vi "get User Info List.vi"(8 "error in (no error)":errorcluster, 11 "[Data] Userinfo Binary in":refnum<class "[Data] Userinfo Binary.lvclass">) -> (0 "error out":errorcluster, 2 "user info":T1(array[cluster]), 3 "[Data] Userinfo Binary out":refnum<class "[Data] Userinfo Binary.lvclass">)   [LabVIEW 2020, in "[Data] Userinfo Binary.lvclass"]
uses:
  [Data] Userinfo Binary.lvclass
  [Data] Userinfo Binary.lvclass/[Data] Userinfo Binary.ctl
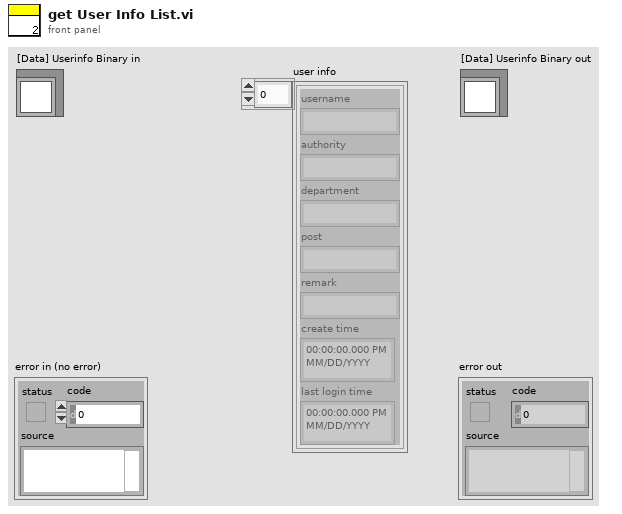
[diagram p1: front panel]
types:
  T1 = cluster{"username":string, "authority":string, "department":string, "post":string, "remark":string, "create time":timestamp, "last login time":timestamp}[]
  T2 = cluster{"username":string, "authority":string, "department":string, "post":string, "remark":string, "create time":timestamp, "last login time":timestamp}
  T3 = typedef "[Data] Userinfo Binary.lvclass/user info.ctl" = cluster{"password":string, "authority":i8, "department":string, "post":string, "remark":string, "create time":timestamp, "last login time":timestamp}
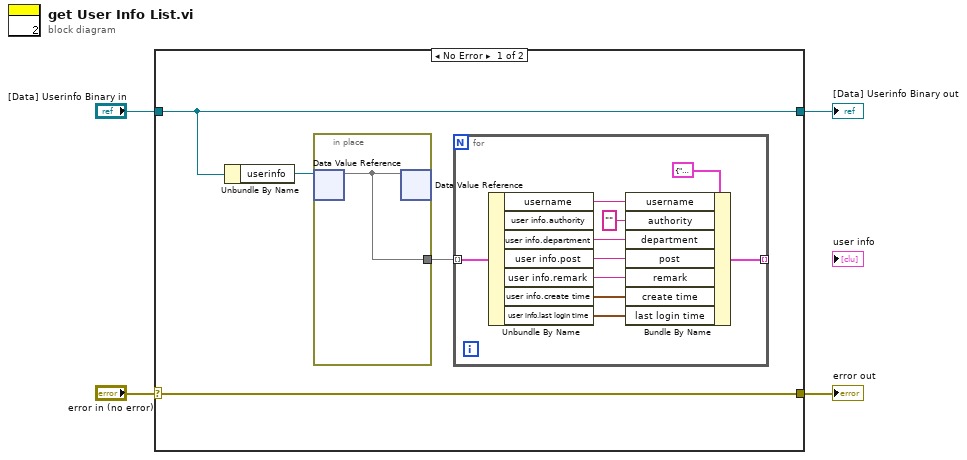
[diagram p0: block diagram]
diagram:
  n1 = case shown="No Error" "error in (no error)" {
    selector: "error in (no error)" -> [w8 w21]
    tunnel: [w8 w21] -> w1
    tunnel: "[Data] Userinfo Binary in" -> [w7 w20]
    tunnel: [w7 w20] -> w3
    frame No Error {
      n2 = Unbundle By Name(w7) -> ("userinfo"=w6:refnum<data-value>)
      n3 = in-place {
        in-place-border: [w19] -> w5
        n4 = in-place-dvr #1(w6) -> (w19:map{string, T3})  [unwired: 1 out]
        n5 = in-place-dvr #1(w19) -> ()  [unwired: 2 out]
      }
      n6 = for {
        tunnel: w5 -> [w18] mode=indexing
        tunnel: [w11] -> _ mode=indexing
        n7 = Unbundle By Name(w18) -> ("username"=w17:string, "user info.department"=w16:string, "user info.post"=w15:string, "user info.remark"=w14:string, "user info.create time"=w13:timestamp, "user info.last login time"=w12:timestamp)  [unwired: 1 out]
        n8 = Bundle By Name(cluster=T2 {"username"="admin", "authority"="", "department"="", "post"="", "remark"="", "create time"=timestamp(3808709554.2178783 s since 1904-01-01), "last login time"=timestamp(3808709806.919703 s since 1904-01-01)} ("user info"), "username"=w17, "authority"="", "department"=w16, "post"=w15, "remark"=w14, "create time"=w13, "last login time"=w12) -> (w11:T2)
      }
    }
    frame Error {
    }
  }
  "error out" <- w1
  "[Data] Userinfo Binary out" <- w3
